vi "Real Transpose Matrix.vi"(11 "Input Matrix":T1) -> (0 "error":i32, 3 "Matrix Transpose":T1)   [LabVIEW 2014, in "NI_AALPro.lvlib"]
doc: "Transposes <B>Input Matrix</B>. If <B>Input Matrix</B> is a complex matrix, the VI performs conjugate transposition. Wire data to the <B>Input Matrix</B> input to determine the polymorphic instance to use or manually select the instance."
uses:
  NI_AALPro.lvlib
  RealMatrix.ctl
  lvanlys.dll
  NI_Matrix.lvlib
panel:
  # "Real Transpose Matrix"
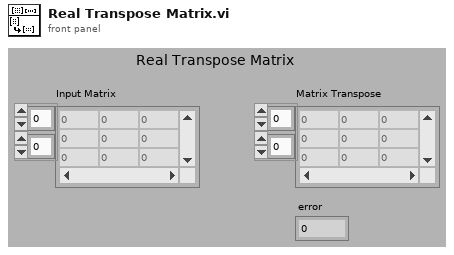
[diagram p1: front panel]
types:
  T1 = typedef "NI_Matrix.lvlib/RealMatrix.ctl" = dbl[][]
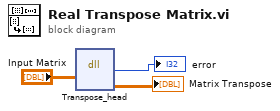
[diagram p0: block diagram]
diagram:
  n1 = dll-call lib="C:/Program Files (x86)/National Instruments/LabVIEW 2014/resource/lvanlys.*" fn="Transpose_head"("Input Matrix"="Input Matrix") -> (→"error":i32, "Matrix Transpose"=→"Matrix Transpose":T1)  [unwired: 5 in, 2 out]
